vi "Global_bypass_ResMeter.vi"() -> ()   [LabVIEW 2019]
panel:
  out "Bypass res meter":bool
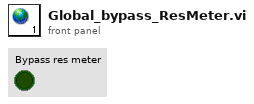
[diagram p1: front panel]
diagram:
